vi "Instalacion_1.vi"() -> ()   [LabVIEW 2025]
panel:
  out "input":string
  out "output":string
  out "Progreso":u8(slide) scale=0.0..80.0
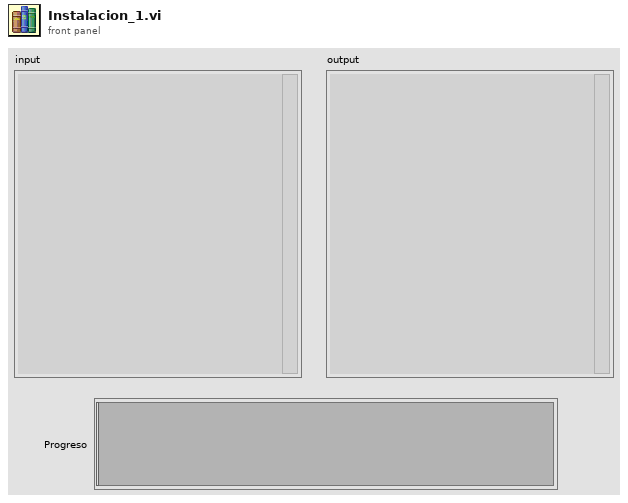
[diagram p1: front panel]
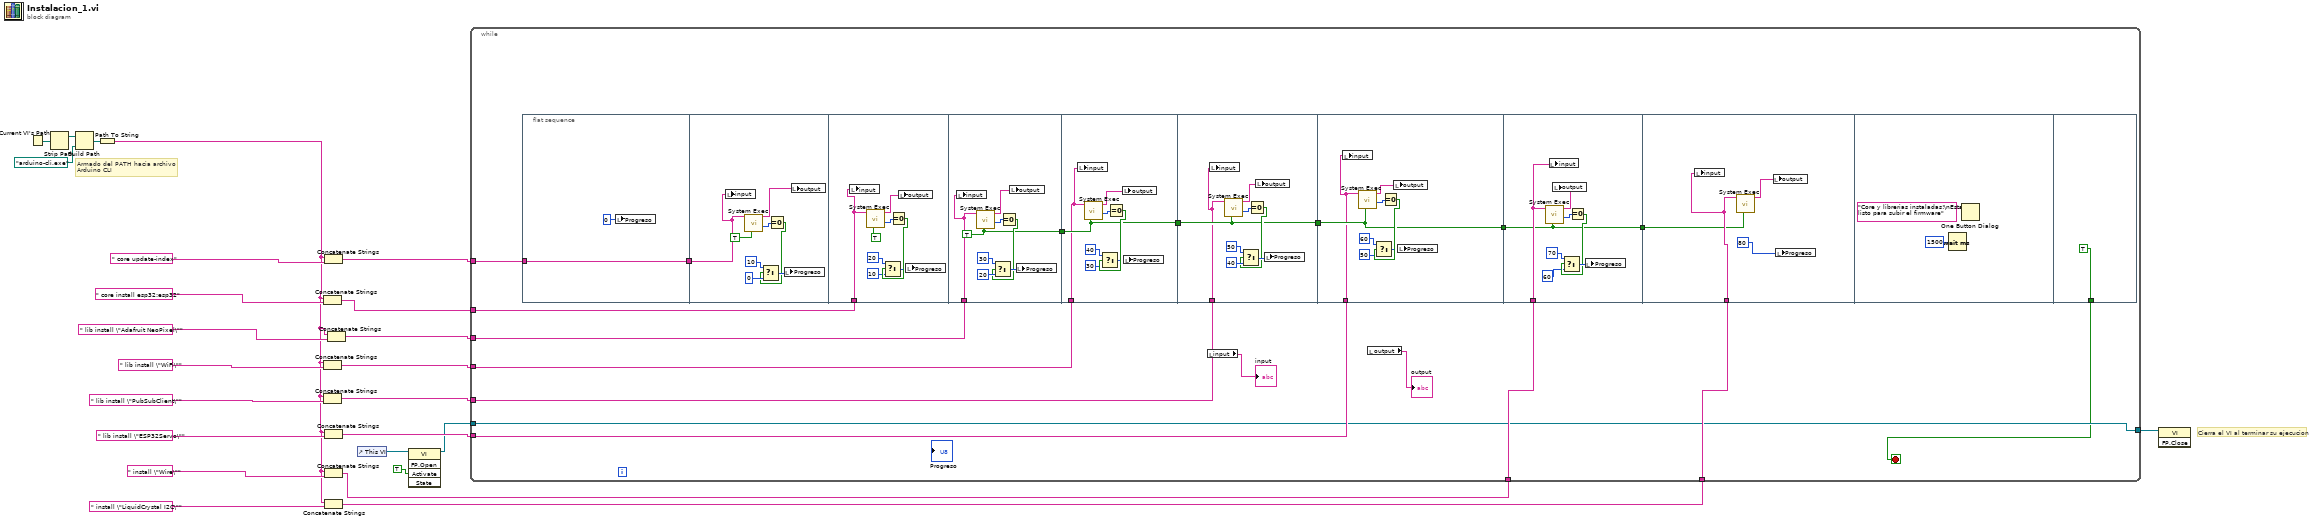
[diagram p0: block diagram]
diagram:
  # "Cierra el VI al terminar su ejecucion"
  # "Armado del PATH hacia archivo \nArduino CLI"
  n1 = Current VI's Path() -> (path=w25:path)
  n2 = Strip Path(path=w25) -> (stripped path=w23:path)  [unwired: 1 out]
  n3 = Build Path(base path=w23, name or relative path=path "arduino-cli.exe") -> (appended path=w21:path)
  n4 = Path To String(path=w21) -> (string=w13:string)
  n5 = Concatenate Strings(w13, " core install esp32:esp32" ("string")) -> (w11:string)
  n6 = Concatenate Strings(w13, " lib install \"WiFi\"" ("string")) -> (w9:string)
  n7 = Concatenate Strings(w13, " lib install \"PubSubClient\"" ("string")) -> (w8:string)
  n8 = Concatenate Strings(w13, " core update-index" ("string")) -> (w12:string)
  n9 = Concatenate Strings(w13, " lib install \"ESP32Servo\"" ("string")) -> (w7:string)
  n10 = Concatenate Strings(w13, " install \"Wire\"" ("string")) -> (w6:string)
  n11 = Concatenate Strings(w13, " install \"LiquidCrystal I2C\"" ("string")) -> (w5:string)
  n12 = Concatenate Strings(w13, " lib install \"Adafruit NeoPixel\"" ("string")) -> (w10:string)
  n13 = control-ref of="This VI"() -> (w4:refnum<vi>)
  n14 = invoke class="VI" method="FP.Open"(reference=w4, "Activate"=TRUE ("Activate?")) -> (reference out=w1:refnum<vi>)  [unwired: 3 in, 4 out]
  n15 = while {
    tunnel: w12 -> [w43]
    tunnel: w11 -> [w42]
    tunnel: w10 -> [w41]
    tunnel: w9 -> [w40]
    tunnel: w8 -> [w39]
    tunnel: w7 -> [w38]
    tunnel: w6 -> [w37]
    tunnel: w5 -> [w36]
    tunnel: [w28] -> w2
    tunnel: w1 -> [w28]
    stop <- w26 stop-if-true
    n16 = flat-sequence {
      tunnel: w43 -> [w45]
      tunnel: [w45] -> w29
      tunnel: w29 -> [w46]
      tunnel: w42 -> [w54]
      tunnel: w41 -> [w62]
      tunnel: [w64] -> w35
      tunnel: w40 -> [w70]
      tunnel: w35 -> [w72]
      tunnel: [w72] -> w34
      tunnel: w39 -> [w78]
      tunnel: w34 -> [w80]
      tunnel: [w80] -> w33
      tunnel: w38 -> [w86]
      tunnel: w33 -> [w88]
      tunnel: [w88] -> w32
      tunnel: w37 -> [w95]
      tunnel: w32 -> [w94]
      tunnel: [w94] -> w27
      tunnel: w36 -> [w104]
      tunnel: w27 -> [w102]
      tunnel: [TRUE ("stop? (T)")] -> w26
      frame #0 {
        n17 = local write "Progreso"(u8 0 ("Progreso")) -> ()
      }
      frame #1 {
        n18 = local write "input"(w46) -> ()
        n19 = call <vilib>:"System Exec.vi"("run minimized? (F)"=TRUE, "command line"=w46) -> ("return code"=w53:i32, "standard output"=w47:string)  [unwired: 6 in, 2 out]
        n20 = Equal To 0?(x=w53) -> (x = 0?=w49:bool)
        n21 = Select(t=10, s=w49, f=0) -> (s? t:f=w50:i32)
        n22 = local write "Progreso"(w50) -> ()
        n23 = local write "output"(w47) -> ()
      }
      frame #2 {
        n24 = local write "input"(w54) -> ()
        n25 = call <vilib>:"System Exec.vi"("run minimized? (F)"=TRUE, "command line"=w54) -> ("return code"=w57:i32, "standard output"=w55:string)  [unwired: 6 in, 2 out]
        n26 = Equal To 0?(x=w57) -> (x = 0?=w61:bool)
        n27 = Select(t=20, s=w61, f=10) -> (s? t:f=w60:i32)
        n28 = local write "output"(w55) -> ()
        n29 = local write "Progreso"(w60) -> ()
      }
      frame #3 {
        w64 = TRUE ("run minimized? (F)")
        n30 = local write "input"(w62) -> ()
        n31 = call <vilib>:"System Exec.vi"("run minimized? (F)"=w64, "command line"=w62) -> ("return code"=w69:i32, "standard output"=w63:string)  [unwired: 6 in, 2 out]
        n32 = Equal To 0?(x=w69) -> (x = 0?=w65:bool)
        n33 = Select(t=30, s=w65, f=20) -> (s? t:f=w66:i32)
        n34 = local write "output"(w63) -> ()
        n35 = local write "Progreso"(w66) -> ()
      }
      frame #4 {
        n36 = local write "input"(w70) -> ()
        n37 = call <vilib>:"System Exec.vi"("run minimized? (F)"=w72, "command line"=w70) -> ("return code"=w73:i32, "standard output"=w71:string)  [unwired: 6 in, 2 out]
        n38 = Equal To 0?(x=w73) -> (x = 0?=w77:bool)
        n39 = Select(t=40, s=w77, f=30) -> (s? t:f=w76:i32)
        n40 = local write "output"(w71) -> ()
        n41 = local write "Progreso"(w76) -> ()
      }
      frame #5 {
        n42 = local write "input"(w78) -> ()
        n43 = call <vilib>:"System Exec.vi"("run minimized? (F)"=w80, "command line"=w78) -> ("return code"=w85:i32, "standard output"=w79:string)  [unwired: 6 in, 2 out]
        n44 = Equal To 0?(x=w85) -> (x = 0?=w81:bool)
        n45 = Select(t=50, s=w81, f=40) -> (s? t:f=w82:i32)
        n46 = local write "output"(w79) -> ()
        n47 = local write "Progreso"(w82) -> ()
      }
      frame #6 {
        n48 = local write "input"(w86) -> ()
        n49 = call <vilib>:"System Exec.vi"("run minimized? (F)"=w88, "command line"=w86) -> ("return code"=w89:i32, "standard output"=w87:string)  [unwired: 6 in, 2 out]
        n50 = Equal To 0?(x=w89) -> (x = 0?=w93:bool)
        n51 = Select(t=60, s=w93, f=50) -> (s? t:f=w92:i32)
        n52 = local write "output"(w87) -> ()
        n53 = local write "Progreso"(w92) -> ()
      }
      frame #7 {
        n54 = call <vilib>:"System Exec.vi"("run minimized? (F)"=w94, "command line"=w95) -> ("return code"=w101:i32, "standard output"=w96:string)  [unwired: 6 in, 2 out]
        n55 = local write "input"(w95) -> ()
        n56 = local write "output"(w96) -> ()
        n57 = Equal To 0?(x=w101) -> (x = 0?=w98:bool)
        n58 = Select(t=70, s=w98, f=60) -> (s? t:f=w99:i32)
        n59 = local write "Progreso"(w99) -> ()
      }
      frame #8 {
        n60 = local write "input"(w104) -> ()
        n61 = call <vilib>:"System Exec.vi"("run minimized? (F)"=w102, "command line"=w104) -> ("standard output"=w105:string)  [unwired: 6 in, 3 out]
        n62 = local write "output"(w105) -> ()
        n63 = local write "Progreso"(80 ("t")) -> ()
      }
      frame #9 {
        n64 = Wait (ms)(milliseconds to wait=u32 1500) -> ()  [unwired: 1 out]
        n65 = One Button Dialog(message="Core y librerias instaladas!\nEsta listo para subir el firmware") -> ()  [unwired: 1 in, 1 out]
      }
      frame #10 {
      }
    }
    n66 = local read "input"() -> (→"input":string)
    n67 = local read "output"() -> (→"output":string)
  }
  n68 = invoke class="VI" method="FP.Close"(reference=w2) -> ()  [unwired: 2 in, 3 out]
